vi "Current Read Array.vi"(8 "error in":errorcluster, 11 "Device in":refnum<class "Device.lvclass">) -> (0 "error out":errorcluster, 2 "Current.SP":dbl[](array[numeric]), 3 "Device out":refnum<class "Device.lvclass">)   [LabVIEW 2023, in "Device.lvclass"]
uses:
  Device.lvclass
  Device.lvclass/Device.ctl
  Low Level Capabilities/Current/Current Setpoint/Current Setpoint.lvclass
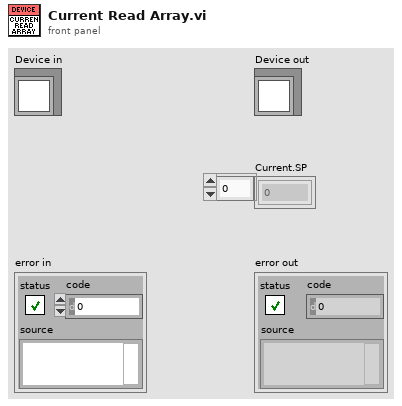
[diagram p1: front panel]
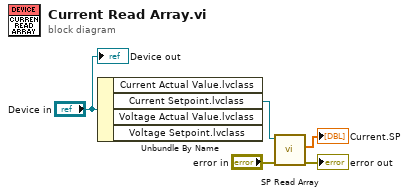
[diagram p0: block diagram]
diagram:
  n1 = Unbundle By Name("Device in") -> ("Current Setpoint.lvclass"=w4:refnum<class "Current Setpoint.lvclass">)  [unwired: 3 out]
  n2 = call-dynamic "SP Read Array.vi"("error in"="error in", "Current Setpoint in"=w4) -> ("error out"=→"error out":errorcluster, "Current SP"=→"Current.SP":dbl[])  [unwired: 6 in, 2 out]
  "Device out" <- "Device in"
